vi "WriteChannel.vi"(4 "Value":bool, 5 "Channel":i32, 6 "error in":errorcluster) -> (0 "error out":errorcluster)   [LabVIEW 2014]
doc: "Write value to the specified channel. The channel must be configured as an output before calling this VI."
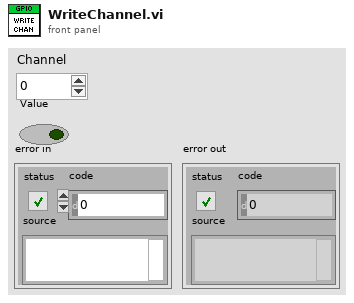
[diagram p1: front panel]
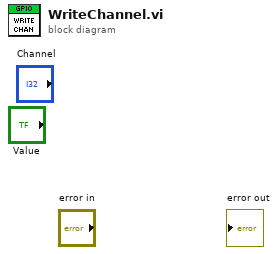
[diagram p0: block diagram]
diagram:
